vi "TEST - AI USB4704 (3) v6.vi"() -> (1 "Graph 1":dynamicdata(graph), 2 "Graph 2":dynamicdata(graph), 3 "Graph 3":dynamicdata(graph), 10 "loop time":dbl format="%.6g", 15 "error array":errorcluster[](array[cluster]))   [LabVIEW 2013]
panel:
  in  "Stop Button":bool
  in  "AI (STOP)":bool
  in  "SAMPLES":dbl
  in  "RATE(Hz)":dbl
  in  "Tab Control":enum32{"Page 1", "Page 2", "Page 3"}(tab)
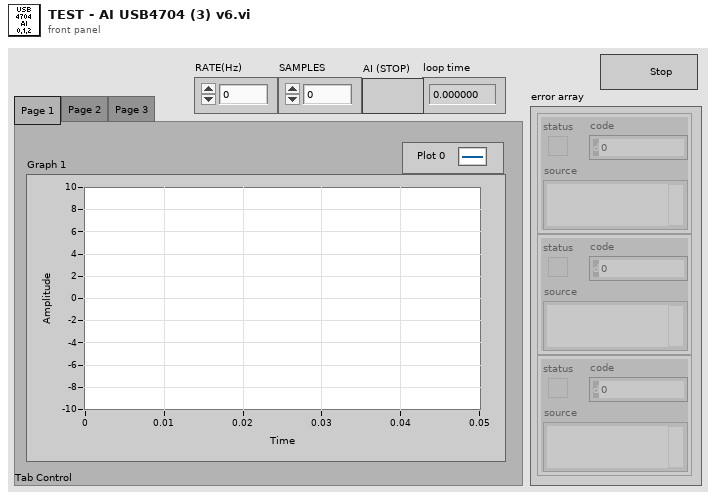
[diagram p1: front panel]
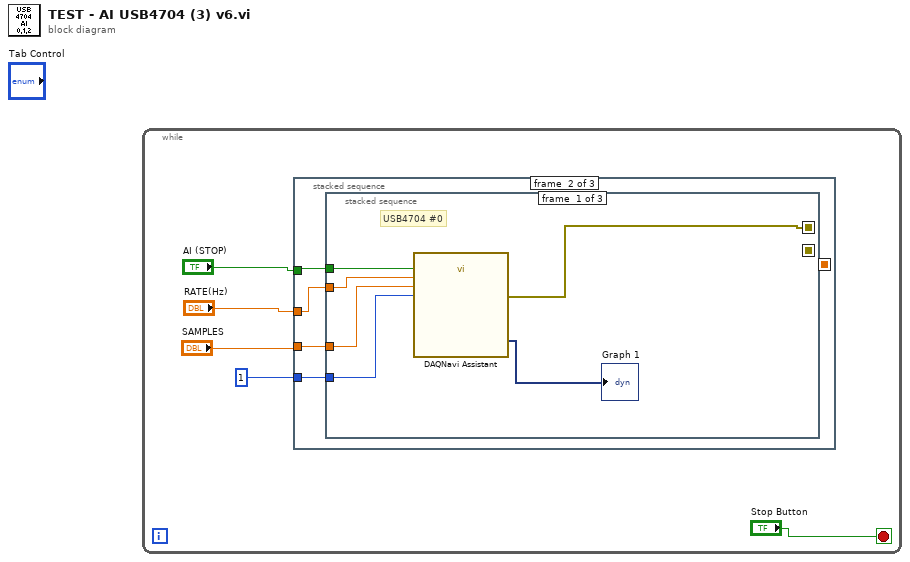
[diagram p0: block diagram]
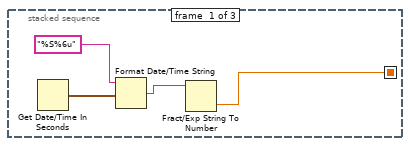
[diagram p2: hidden frame]
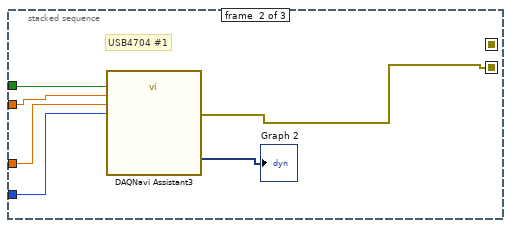
[diagram p3: hidden frame]
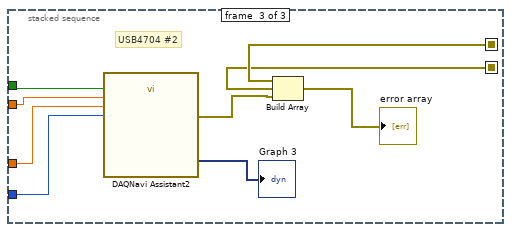
[diagram p4: hidden frame]
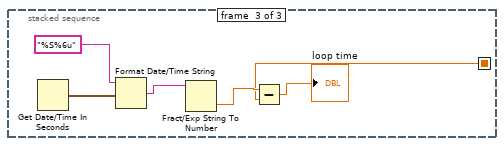
[diagram p5: hidden frame]
diagram:
  n1 = while {
    stop <- "Stop Button" stop-if-true
    n2 = stacked-sequence {
      seq-local: [w6 _ _] -> [_ _ w36]
      tunnel: "AI (STOP)" -> [_ w13 _]
      tunnel: 1 -> [_ w10 _]
      tunnel: "RATE(Hz)" -> [_ w12 _]
      tunnel: "SAMPLES" -> [_ w11 _]
      frame #0 {
        n3 = Get Date/Time In Seconds() -> (seconds since 1Jan1904=w8:timestamp)
        n4 = Format Date/Time String(time format string (%c)="%S%6u", seconds (now)=w8) -> (date/time string=w7:string)  [unwired: 1 in]
        n5 = Fract/Exp String To Number(string=w7) -> (number=w6:dbl)  [unwired: 3 in, 1 out]
      }
      frame #1 {
        n6 = stacked-sequence {
          seq-local: [w14 _ _] -> [_ _ w29]
          seq-local: [_ w20 _] -> [_ _ w28]
          tunnel: w13 -> [w18 w25 w34]
          tunnel: w12 -> [w17 w24 w33]
          tunnel: w11 -> [w16 w23 w32]
          tunnel: w10 -> [w15 w22 w31]
          frame #0 {
            # "USB4704 #0"
            n7 = call "DAQNavi Assistant"("stop(true)"=w18, "conversion rate(Hz)"=w17, "samples"=w16, "time out(10s)"=w15) -> ("error out"=w14:errorcluster, "data out(DDT)"=→"Graph 1":dynamicdata)  [unwired: 22 in]
          }
          frame #1 {
            # "USB4704 #1"
            n8 = call "DAQNavi Assistant3"("stop(true)"=w25, "conversion rate(Hz)"=w24, "samples"=w23, "time out(10s)"=w22) -> ("error out"=w20:errorcluster, "data out(DDT)"=→"Graph 2":dynamicdata)  [unwired: 22 in]
          }
          frame #2 {
            # "USB4704 #2"
            n9 = call "DAQNavi Assistant2"("stop(true)"=w34, "conversion rate(Hz)"=w33, "samples"=w32, "time out(10s)"=w31) -> ("error out"=w27:errorcluster, "data out(DDT)"=→"Graph 3":dynamicdata)  [unwired: 22 in]
            n10 = Build Array(w29, w28, w27) -> (→"error array":errorcluster[])
          }
        }
      }
      frame #2 {
        n11 = Get Date/Time In Seconds() -> (seconds since 1Jan1904=w39:timestamp)
        n12 = Format Date/Time String(time format string (%c)="%S%6u", seconds (now)=w39) -> (date/time string=w38:string)  [unwired: 1 in]
        n13 = Fract/Exp String To Number(string=w38) -> (number=w37:dbl)  [unwired: 3 in, 1 out]
        n14 = Subtract(x=w37, y=w36) -> (x-y=→"loop time":dbl)
      }
    }
  }
